vi "SendToDb.vi"(0 "reference in":refnum<class "DO.lvclass">, 11 "error in (no error)":errorcluster) -> (4 "reference out":refnum<class "DO.lvclass">, 15 "error out":errorcluster)   [LabVIEW 2019, in "DO.lvclass"]
uses:
  DO.lvclass
  D:/GIT H4000/H4000/src/Proccess_class/Proccess.lvclass
  Proccess_class/Proccess.lvclass/Proccess.ctl
  DO.lvclass/DO.ctl
  TypeDef/AlarmType.ctl
  Logger_class/EventType.ctl
  Logger_class/EventData.ctl
  Logger_class/Logger.lvclass
  Proccess_class/Proccess.lvclass
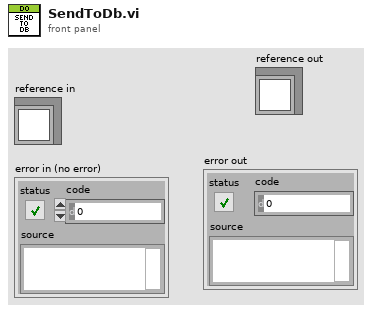
[diagram p1: front panel]
types:
  T1 = typedef "AlarmType.ctl" = enum16{"Normal", "Warning", "Alarm"}
  T2 = typedef "Logger.lvclass/EventType.ctl" = enum16{"DI", "DO", "DA", "AI", "AO", "AA", "CMD", "ERR", "ST"}
  T3 = typedef "Logger.lvclass/EventData.ctl" = cluster{"obj_tag":string, "event_tag":string, "Description":string, "EVENT TYPE":T2, "ALARM TYPE":T1, "Value DBL":dbl, "Value INT":i32, "Value STR":string, "Time Stamp":timestamp}
  T4 = typedef "Proccess.lvclass/TAGs.ctl" = cluster{"TAG":string, "PTAG":string, "DESC":string}
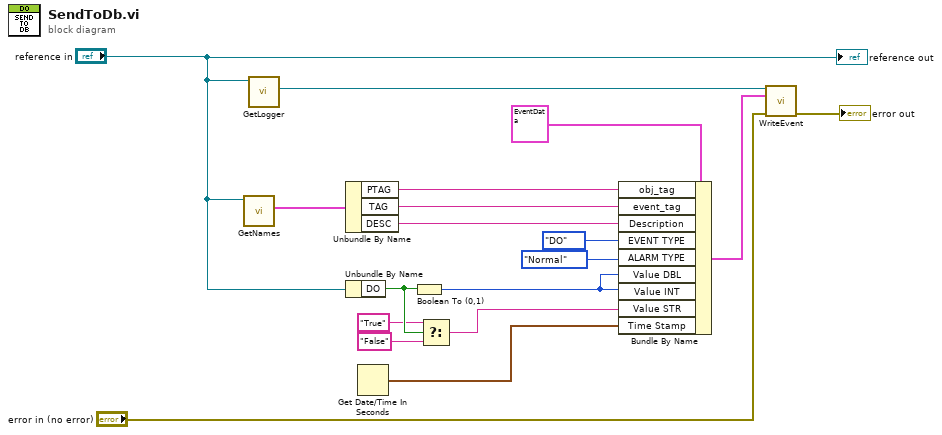
[diagram p0: block diagram]
diagram:
  n1 = call "GetNames.vi"("Proccess in"="reference in") -> ("Tags"=w12:T4)  [unwired: 10 in]
  n2 = call "GetLogger.vi"("Proccess in"="reference in") -> ("Logger"=w14:refnum<class "Logger.lvclass">)  [unwired: 10 in]
  n3 = Unbundle By Name(w12) -> ("PTAG"=w11:string, "TAG"=w10:string, "DESC"=w9:string)
  n4 = Unbundle By Name("reference in") -> ("DO"=w5:bool)
  n5 = Get Date/Time In Seconds() -> (seconds since 1Jan1904=w1:timestamp)
  n6 = Boolean To (0,1)(Boolean=w5) -> (0, 1=w6:i16)
  n7 = Select(t="True" ("Value STR"), s=w5, f="False" ("Value STR")) -> (s? t:f=w2:string)
  n8 = Bundle By Name(cluster=T3 {"obj_tag"="", "event_tag"="", "Description"="", "EVENT TYPE"=enum."AO", "ALARM TYPE"=enum."Alarm", "Value DBL"=0.0, "Value INT"=0, "Value STR"="", "Time Stamp"=timestamp(0 s since 1904-01-01)} ("Event"), "obj_tag"=w11, "event_tag"=w10, "Description"=w9, "EVENT TYPE"=EventType."DO", "ALARM TYPE"=AlarmType."Normal", "Value DBL"=w6, "Value INT"=w6, "Value STR"=w2, "Time Stamp"=w1) -> (w16:T3)
  n9 = call "WriteEvent.vi"("reference in"=w14, "Event"=w16, "error in (no error)"="error in (no error)") -> ("error out"=→"error out":errorcluster)  [unwired: 11 in, 1 out]
  "reference out" <- "reference in"
